vi "MotorCalc.vi"(6 "l3":dbl, 7 "Pd":T1, 8 "l2":dbl, 9 "l1":dbl, 10 "leg":dbl=0.088, 11 "crank":dbl=0.03) -> (1 "m3":dbl, 2 "m2":dbl, 3 "m1":dbl)   [LabVIEW 2019]
uses:
  <vilib>/Analysis/Matrix/Datatypes/RealMatrix.ctl
  <vilib>/Analysis/Matrix/NI_Matrix.lvlib
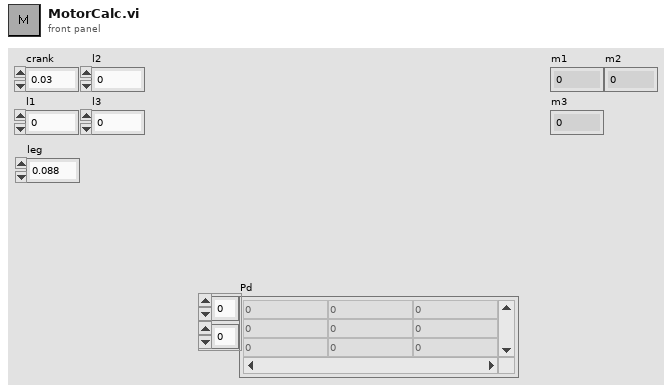
[diagram p1: front panel]
types:
  T1 = typedef "NI_Matrix.lvlib/RealMatrix.ctl" = dbl[][]
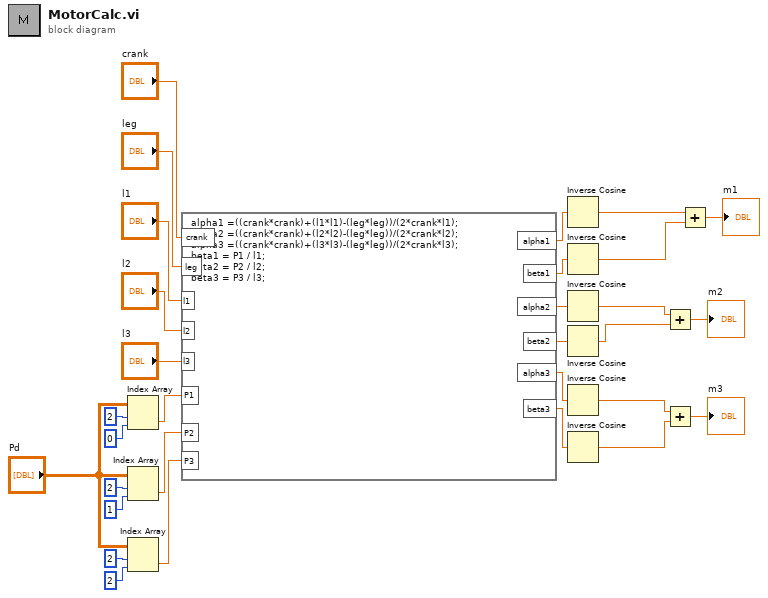
[diagram p0: block diagram]
diagram:
  n1 = Index Array(array="Pd", index (row)=2, index (col)=0) -> (element=w18:dbl)
  n2 = Index Array(array="Pd", index (row)=2, index (col)=1) -> (element=w17:dbl)
  n3 = Index Array(array="Pd", index (row)=2, index (col)=2) -> (element=w16:dbl)
  n4 = formula code="alpha1 =((crank*crank)+(l1*l1)-(leg*leg))/(2*crank*l1);\nalpha2 =((crank*crank)+(l2*l2)-(leg*leg))/(2*crank*l2);\nalpha3 =((crank*crank)+(l3*l3)-(leg*leg))/(2*crank*l3);\nbeta1 = P1 / l1;\nbeta2 = P2 / l2;\nbeta3 = P3 / l3;"("crank"="crank", "leg"="leg", "l1"="l1", "l2"="l2", "l3"="l3", "P1"=w18, "P2"=w17, "P3"=w16) -> ("alpha1"=w10:dbl, "alpha2"=w12:dbl, "alpha3"=w14:dbl, "beta1"=w11:dbl, "beta2"=w13:dbl, "beta3"=w15:dbl)
  n5 = Inverse Cosine(1:w10) -> (0:w9:dbl)
  n6 = Inverse Cosine(1:w11) -> (0:w8:dbl)
  n7 = Inverse Cosine(1:w12) -> (0:w5:dbl)
  n8 = Inverse Cosine(1:w13) -> (0:w4:dbl)
  n9 = Inverse Cosine(1:w14) -> (0:w7:dbl)
  n10 = Inverse Cosine(1:w15) -> (0:w6:dbl)
  n11 = Add(x=w5, y=w4) -> (x+y=→"m2":dbl)
  n12 = Add(x=w7, y=w6) -> (x+y=→"m3":dbl)
  n13 = Add(x=w9, y=w8) -> (x+y=→"m1":dbl)
